vi "Parse Cluster Configuration.vi"(8 "error in (no error)":errorcluster, 10 "Cluster in":variant, 11 "Register Name in":string) -> (0 "error out":errorcluster, 2 "Cluster Configuration":T1)   [LabVIEW 2018, in "Scalar IO Operations.lvlib"]
uses:
  Scalar IO Operations.lvlib
  TypeDefs/Cluster Configuration.ctl
  <vilib>/Utility/Data Type/Type Definitions/Data Type.ctl
  TypeDefs/Cluster Configuration Store.ctl
  TypeDefs/FXP Configuration.ctl
  <vilib>/fxp/LVFixedPointRepBitsTypeDef.ctl
  <vilib>/fxp/LVFixedPointRepRangeTypeDef.ctl
  <vilib>/Utility/Data Type/NI_Data Type.lvlib
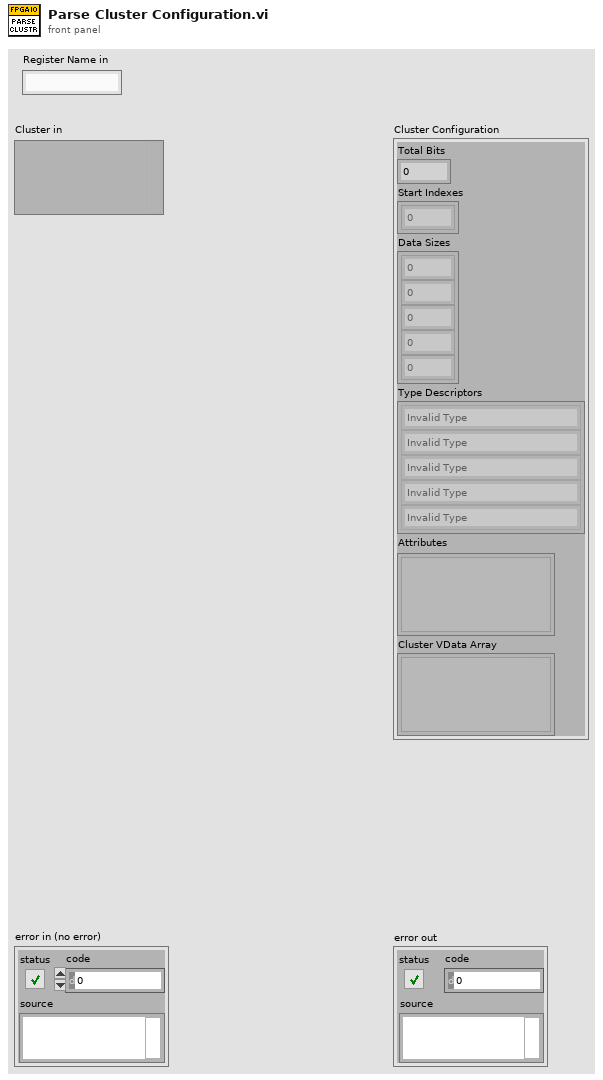
[diagram p1: front panel]
types:
  T1 = typedef "Scalar IO Operations.lvlib/Cluster Configuration.ctl" = cluster{"Total Bits":i32, "Start Indexes":i32[], "Data Sizes":i32[], "Type Descriptors":T2[], "Attributes":variant[], "Cluster VData Array":variant[]}
  T2 = typedef "NI_Data Type.lvlib/Data Type.ctl" = enum8{"Invalid Type", "Void", "I8", "I16", "I32", "I64", "U8", "U16", "U32", "U64", "Single Float", "Double Float", "Extended Float", "Single Complex", "Double Complex", "Extended Complex", "Enum U8", "Enum U16", "Enum U32", "Enum U64", "Single Float With Unit", "Double Float With Unit", "Extended Float With Unit", "Single Complex with Unit", "Double Complex with Unit", "Extended Complex with Unit", "Boolean", "String", "Path", "Picture", "Tag", "Array", "Cluster", "Variant", "LV Variant", "Waveform", "Timestamp", "Digital Waveform", "Digital Data", "ExpressData", "Refnum", "External Data", "VI", "Poly VI", "LabVIEW Class Instance", "Fixed Point"}
  T3 = typedef "Scalar IO Operations.lvlib/Cluster Configuration Store.ctl" = cluster{"Register Names":string[], "Cluster Configurations":T1[]}
  T4 = typedef "Scalar IO Operations.lvlib/FXP Configuration.ctl" = cluster{"FXP Representation":T5, "FXP Range":T6}
  T5 = typedef "LVFixedPointRepBitsTypeDef.ctl" = cluster{"Signed":bool, "Word Length":u32, "Integer Word Length":i32}
  T6 = typedef "LVFixedPointRepRangeTypeDef.ctl" = cluster{"Range Min":dbl, "Range Max":dbl, "Delta":dbl}
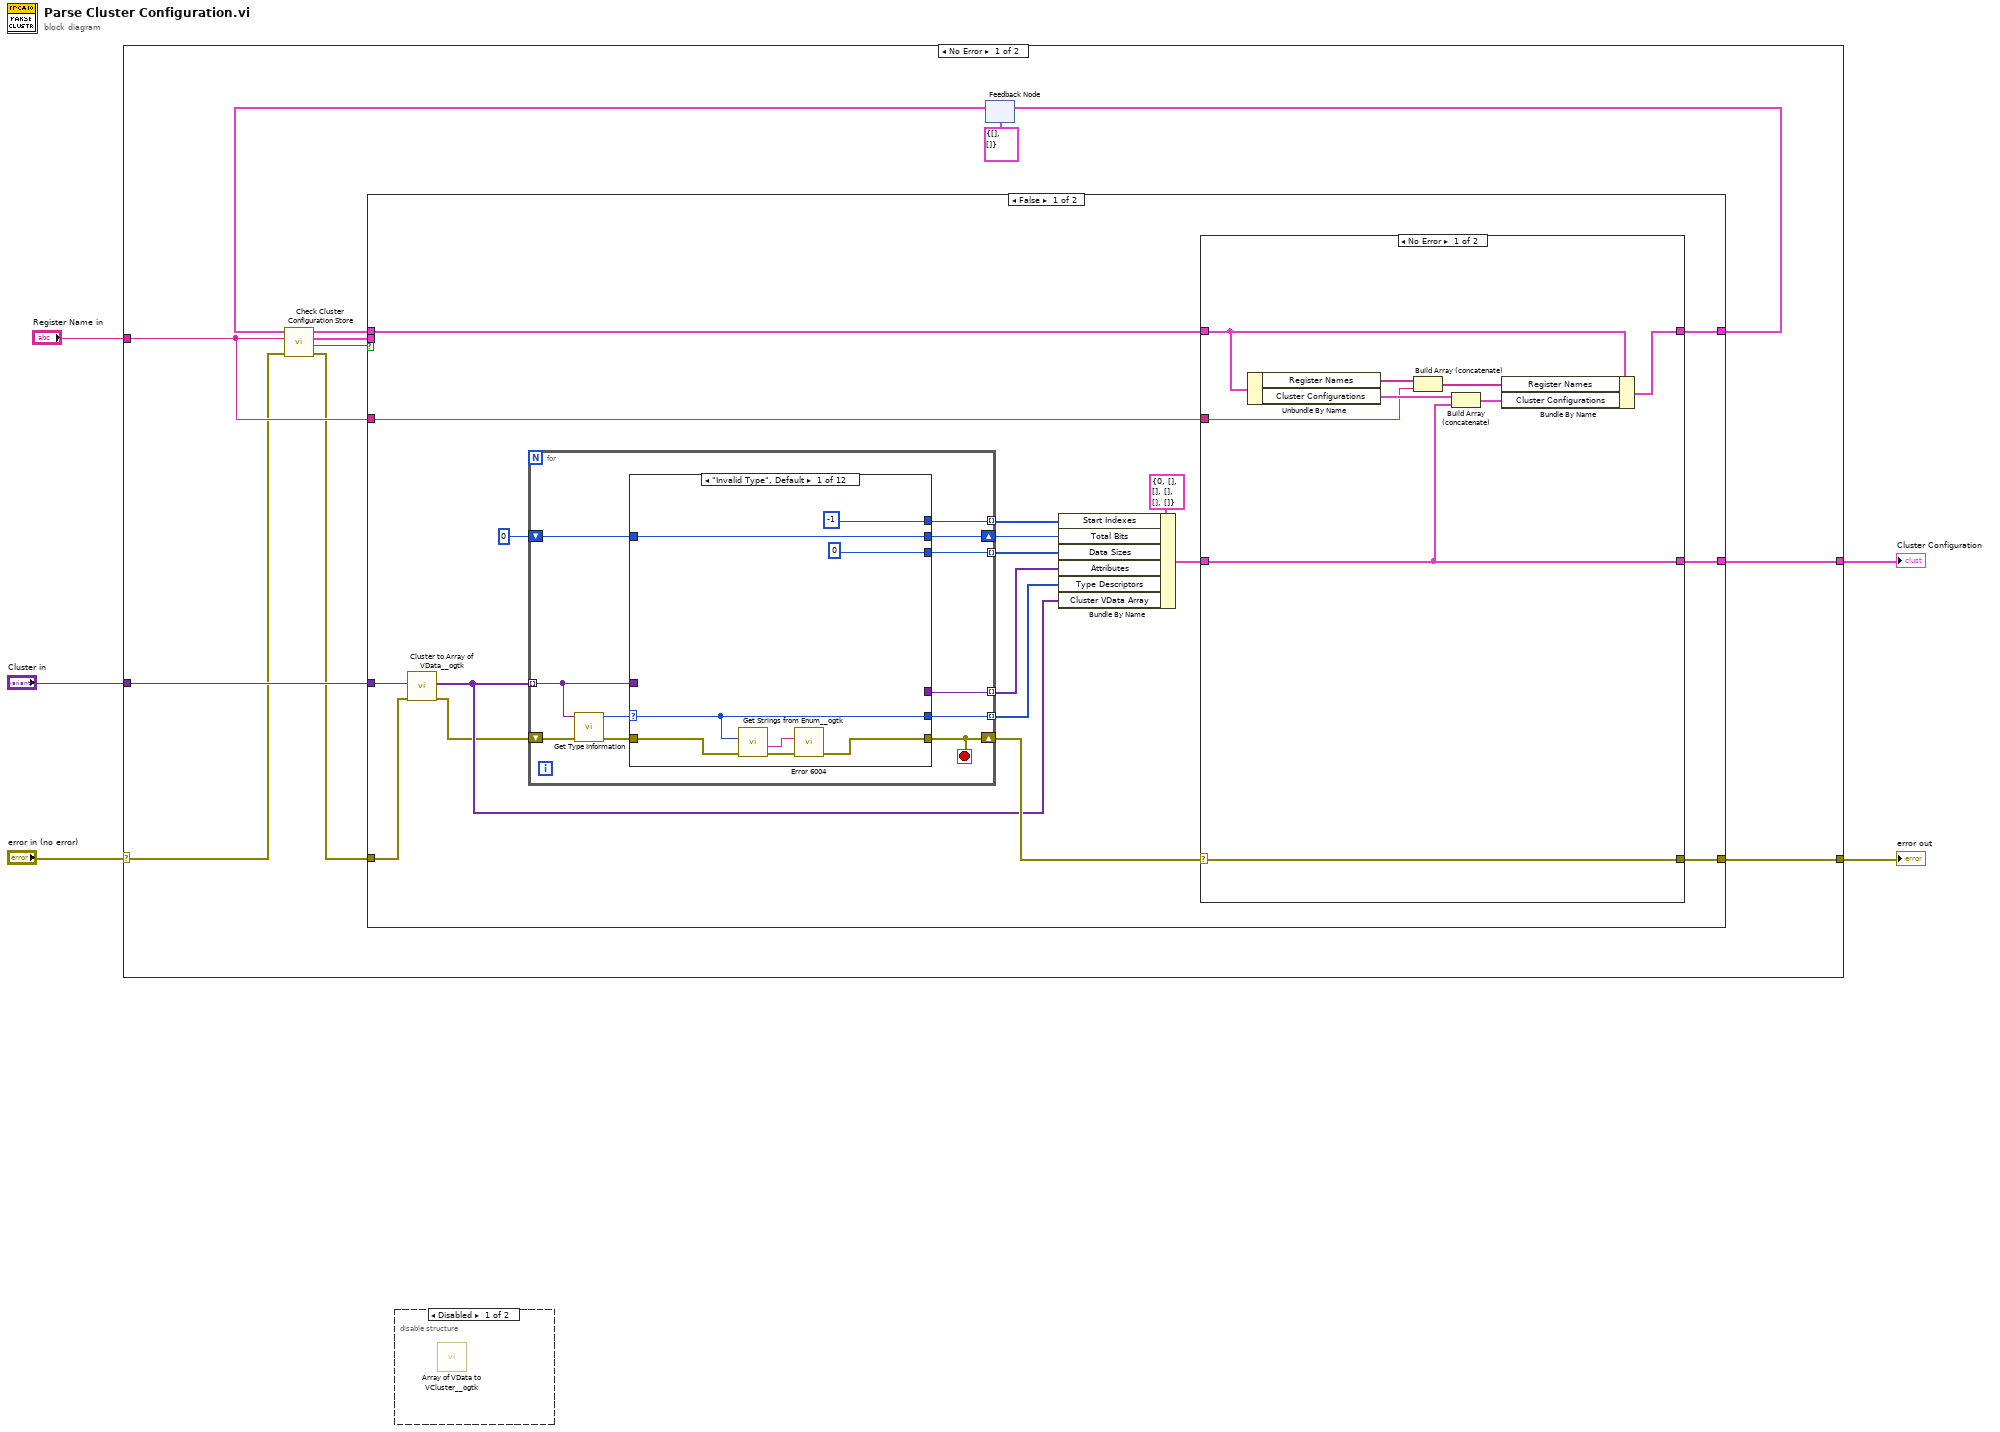
[diagram p0: block diagram]
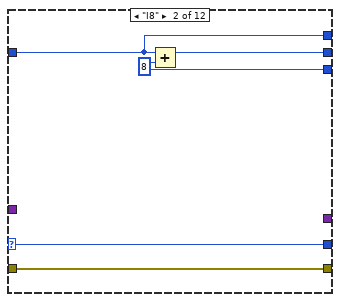
[diagram p3: hidden frame]
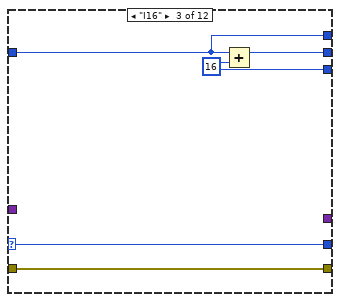
[diagram p4: hidden frame]
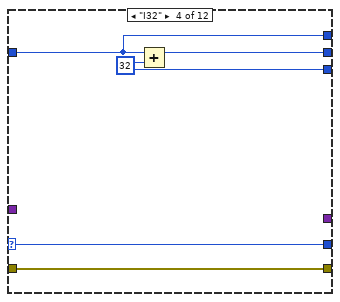
[diagram p5: hidden frame]
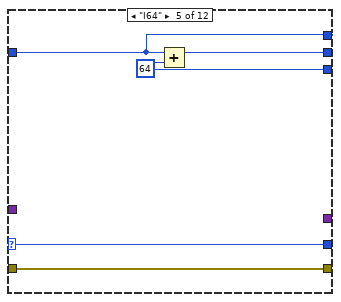
[diagram p6: hidden frame]
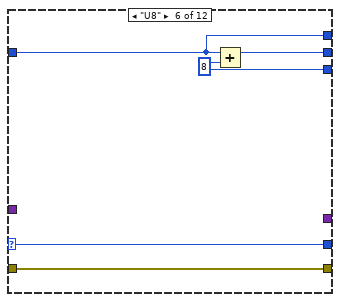
[diagram p7: hidden frame]
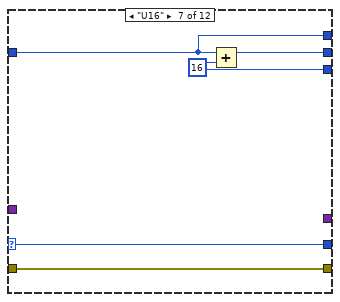
[diagram p8: hidden frame]
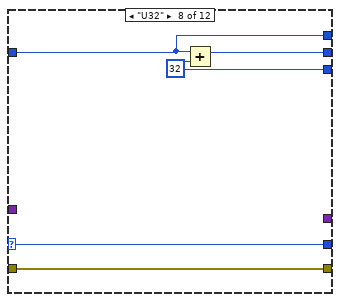
[diagram p9: hidden frame]
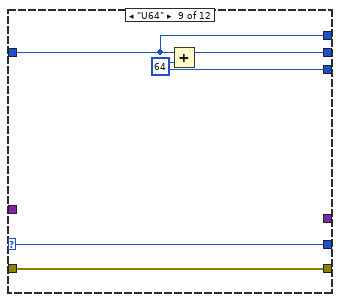
[diagram p10: hidden frame]
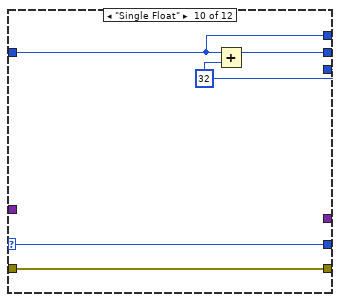
[diagram p11: hidden frame]
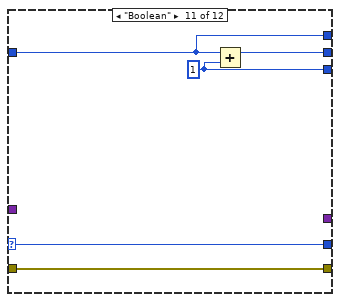
[diagram p12: hidden frame]
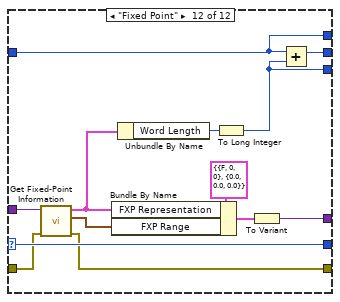
[diagram p13: hidden frame]
diagram:
  n1 = case shown="No Error" "error in (no error)" {
    selector: "error in (no error)" -> [w7 w133]
    tunnel: "Cluster in" -> [w16 _]
    tunnel: [w17 w133] -> w3
    tunnel: "Register Name in" -> [w13 _]
    tunnel: [w8 _] -> w1
    frame No Error {
      n2 = feedback #1(T3 {"Register Names"=[], "Cluster Configurations"=[]} ("Cluster Configuration Store out")) -> (w11:T3)
      n3 = call "Check Cluster Configuration Store.vi"("error in (no error)"=w7, "register name"=w13, "Cluster Configuration Store in"=w11) -> ("error IO"=w6:errorcluster, "Found"=w15:bool, "Cluster Configuration out"=w10:T1, "Cluster Configuration Store out"=w14:T3)  [unwired: 5 in]
      n4 = case shown="False" w15 {
        tunnel: w16 -> [w21 _]
        tunnel: w6 -> [w19 w132]
        tunnel: [w27 w132] -> w17
        tunnel: w14 -> [w25 w131]
        tunnel: w13 -> [w24 _]
        tunnel: [w23 w131] -> w12
        tunnel: w10 -> [_ w130]
        tunnel: [w22 w130] -> w8
        frame False {
          n5 = call <userlib>:"Cluster to Array of VData__ogtk.vi"("error in (no error)"=w19, "Cluster"=w21) -> ("error out"=w18:errorcluster, "Array of VData"=w20:variant[])  [unwired: 8 in]
          n6 = for {
            tunnel: w20 -> [w57] mode=indexing
            shift-right: [w55] -> w33
            shift-left: 0 -> [w56]
            tunnel: [w54] -> w29 mode=indexing
            tunnel: [w53] -> w30 mode=indexing
            tunnel: [w52] -> w32 mode=indexing
            tunnel: [w51] -> w31 mode=indexing
            shift-right: [w48] -> w28
            shift-left: w18 -> [w50]
            stop <- w48 stop-if-true
            n7 = call <vilib>:"Get Type Information.vi"("error in (no error)"=w50, "Variant"=w57) -> ("error out"=w49:errorcluster, "Type"=w58:T2)  [unwired: 5 in, 3 out]
            n8 = case shown="\"Invalid Type\", Default" w58 {
              selector: w58 -> [w61 w69 w74 w79 w84 w89 w94 w99 w104 w109 w114 w125]
              tunnel: w57 -> [_ _ _ _ _ _ _ _ _ _ _ w129]
              tunnel: w56 -> [w66 w70 w75 w80 w85 w90 w95 w100 w105 w110 w115 w126]
              tunnel: [w66 w71 w76 w81 w86 w91 w96 w101 w106 w111 w116 w127] -> w55
              tunnel: [-1 w70 w75 w80 w85 w90 w95 w100 w105 w110 w115 w126] -> w54
              tunnel: [w61 w69 w74 w79 w84 w89 w94 w99 w104 w109 w114 w125] -> w53
              tunnel: [0 ("y") w68 w73 w78 w82 w88 w93 w98 w103 w108 w113 w124] -> w52
              tunnel: [_ _ _ _ _ _ _ _ _ _ _ w119] -> w51
              tunnel: w49 -> [w60 w67 w72 w77 w83 w87 w92 w97 w102 w107 w112 w118]
              tunnel: [w59 w67 w72 w77 w83 w87 w92 w97 w102 w107 w112 w117] -> w48
              frame "Invalid Type", Default {
                n9 = call <userlib>:"Get Strings from Enum__ogtk.vi"("error in (no error)"=w60, "Enum"=w61) -> ("error out"=w62:errorcluster, "String Value"=w63:string)  [unwired: 6 in, 2 out]
                n10 = call "Error 6004.vi"("error in (no error)"=w62, "datatype"=w63) -> ("error out"=w59:errorcluster)  [unwired: 9 in]
              }
              frame "I8" {
                w68 = 8 ("y")
                n11 = Add(x=w70, y=w68) -> (x+y=w71:i32)
              }
              frame "I16" {
                w73 = 16 ("y")
                n12 = Add(x=w75, y=w73) -> (x+y=w76:i32)
              }
              frame "I32" {
                w78 = 32 ("y")
                n13 = Add(x=w80, y=w78) -> (x+y=w81:i32)
              }
              frame "I64" {
                w82 = 64 ("y")
                n14 = Add(x=w85, y=w82) -> (x+y=w86:i32)
              }
              frame "U8" {
                w88 = 8 ("y")
                n15 = Add(x=w90, y=w88) -> (x+y=w91:i32)
              }
              frame "U16" {
                w93 = 16 ("y")
                n16 = Add(x=w95, y=w93) -> (x+y=w96:i32)
              }
              frame "U32" {
                w98 = 32 ("y")
                n17 = Add(x=w100, y=w98) -> (x+y=w101:i32)
              }
              frame "U64" {
                w103 = 64 ("y")
                n18 = Add(x=w105, y=w103) -> (x+y=w106:i32)
              }
              frame "Single Float" {
                w108 = 32 ("y")
                n19 = Add(x=w110, y=w108) -> (x+y=w111:i32)
              }
              frame "Boolean" {
                w113 = 1 ("y")
                n20 = Add(x=w115, y=w113) -> (x+y=w116:i32)
              }
              frame "Fixed Point" {
                n21 = call <vilib>:"Get Fixed-Point Information.vi"("error in (no error)"=w118, "Variant"=w129) -> ("error out"=w117:errorcluster, "FXP Range"=w122:T6, "FXP Representation"=w121:T5)  [unwired: 6 in, 1 out]
                n22 = Bundle By Name(cluster=T4 {"FXP Representation"={"Signed"=FALSE, "Word Length"=0, "Integer Word Length"=0}, "FXP Range"={"Range Min"=0.0, "Range Max"=0.0, "Delta"=0.0}} ("FXP Configuration"), "FXP Representation"=w121, "FXP Range"=w122) -> (w120:T4)
                n23 = Unbundle By Name(w121) -> ("Word Length"=w128:u32)
                n24 = To Long Integer(number=w128) -> (32bit integer=w124:i32)
                n25 = To Variant(anything=w120) -> (Variant=w119:variant)
                n26 = Add(x=w126, y=w124) -> (x+y=w127:i32)
              }
            }
          }
          n27 = Bundle By Name(cluster=T1 {"Total Bits"=0, "Start Indexes"=[], "Data Sizes"=[], "Type Descriptors"=[], "Attributes"=[], "Cluster VData Array"=[]} ("Cluster Configuration"), "Start Indexes"=w29, "Total Bits"=w33, "Data Sizes"=w32, "Attributes"=w31, "Type Descriptors"=w30, "Cluster VData Array"=w20) -> (w26:T1)
          n28 = case shown="No Error" w28 {
            selector: w28 -> [w44 w47]
            tunnel: [w44 w47] -> w27
            tunnel: w26 -> [w36 w45]
            tunnel: w25 -> [w40 w46]
            tunnel: w24 -> [w41 _]
            tunnel: [w37 w46] -> w23
            tunnel: [w36 w45] -> w22
            frame No Error {
              n29 = Unbundle By Name(w40) -> ("Register Names"=w43:string[], "Cluster Configurations"=w42:T1[])
              n30 = Build Array (concatenate)(w43, w41) -> (w39:string[])
              n31 = Build Array (concatenate)(w42, w36) -> (w38:T1[])
              n32 = Bundle By Name(cluster=w40, "Register Names"=w39, "Cluster Configurations"=w38) -> (w37:T3)
            }
            frame Error {
            }
          }
        }
        frame True {
        }
      }
      n33 = feedback-in #1(w12) -> ()
    }
    frame Error {
    }
  }
  "Cluster Configuration" <- w1
  "error out" <- w3
  n34 = disable-structure shown="Disabled" {
    frame Disabled {
      n35 = call <userlib>:"Array of VData to VCluster__ogtk.vi"() -> ()  [unwired: 10 in, 2 out]
    }
    frame Enabled {
    }
  }
